vi "Close cRIO.vi"(6 "Development Environment":bool, 8 "error in (no error)":errorcluster, 11 "FPGA Ref":T1) -> ()   [LabVIEW 2018]
uses:
  Variables/Global - cRIO Configuration Options.vi
  <vilib>/rvi/interface/nirviCloseFPGA/nirviCloseFPGA.xnode
  <vilib>/FPGAPlugInAG/Dynamic/niLvFpga_Close_Dynamic.vi
  FPGA/FPGA VI Reference.ctl
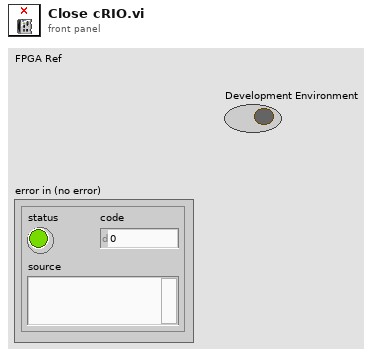
[diagram p1: front panel]
types:
  T1 = typedef "FPGA VI Reference.ctl" = refnum<k20>
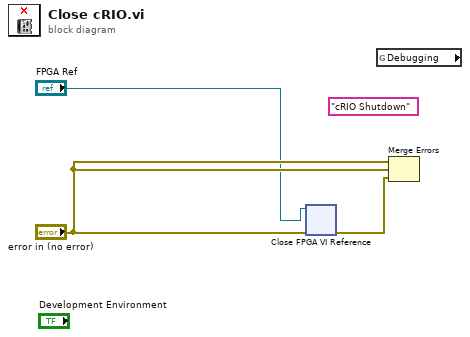
[diagram p0: block diagram]
diagram:
  w4 = "cRIO Shutdown" ("Line to Write(\"\")")
  n1 = xnode "Close FPGA VI Reference"("FPGA VI Reference In"="FPGA Ref", "error in"="error in (no error)") -> ("error out"=w6:errorcluster)
  n2 = global read "Global - cRIO Configuration Options.vi" "Debugging"() -> (w2)
  n3 = Merge Errors("error in (no error)", "error in (no error)", w6) -> ()  [unwired: 1 out]
